vi "Read DSP Reset.vi"(2 "gen":refnum<class "niUSRP Tx DSP v2 FPGA.lvclass">) -> (4 "dsp reset":bool)   [LabVIEW 2025, in "niUSRP Tx DSP v2 FPGA.lvclass"]
doc: "this VI retrieves the dsp.reset signal as configured by the host. a maximum fanour constraint is placed on the signal so that our reset signal does not introduce high fanout nets that lead to Timing Errors (lower compile success rate). this VI should be used to read the reset signal so that all reset signals have the same pipelining applied to them. breaking the timing between resets across the fpga may create undesireable behavior."
uses:
  niUSRP Tx DSP v2 FPGA.lvclass
  niUSRP Tx DSP v2 FPGA.lvclass/niUSRP Tx DSP v2 FPGA.ctl
  <vilib>/rvi/DataTransferAndStorage/Container/Common/niFpgaContainerExecOnDevCompGetState.vi
  <vilib>/rvi/Emulation/niFpgaEmulationIsFPGAContextNoSignature.vi
  <vilib>/rvi/DataTransferAndStorage/Container/Common/niFpgaContainerGetUniqueNameForEmu.vi
  <vilib>/rvi/Memory/Memory_Emulation/niFpgaMemoryEmulationCacheClearOnFirstRun.vi
  <vilib>/rvi/Memory/Memory_Emulation/nirvimemoryEmulationManagerCache_MakeExclusive.vi
  <vilib>/rvi/Memory/Memory_Emulation/niFpgaMemoryEmulationValidateCache.vi
  <vilib>/rvi/Memory/Memory_Emulation/nirvimemoryEmulationManagerCache_InsertValue.vi
  <vilib>/Utility/error.llb/Clear Errors.vi
  <vilib>/rvi/Memory/Memory_Emulation/nirvimemoryEmulationManagerCache_ReleaseExclusive.vi
  <vilib>/rvi/Memory/Memory_Emulation/nirvimemoryEmulationManagerCache_GetValue.vi
  <vilib>/rvi/Memory/Memory_Emulation/nirvimemoryEmulationManagerCache_SetValue.vi
  <vilib>/rvi/Emulation/niFpgaProcessEmulError.vi
  <vilib>/rvi/Emulation/niFpgaSctlEmulationGetInTimedLoop.vi
  <vilib>/rvi/DataTransferAndStorage/Container/XNode/niFpgaContainer.xnode
  <vilib>/rvi/DataTransferAndStorage/Register/Emulation/niFpgaRegisterEmulationRefIn.vi
  <instrlib>/_niInstr/Basic Elements/v1/FPGA/niInstr Basic Elements v1 FPGA.lvlib
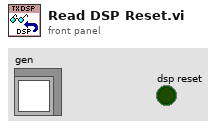
[diagram p1: front panel]
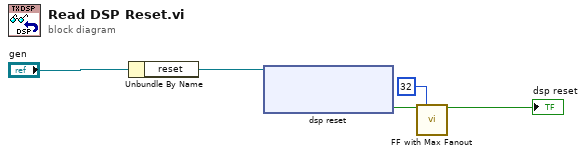
[diagram p0: block diagram]
diagram:
  n1 = Unbundle By Name("gen") -> ("reset"=w4:refnum<k21>)
  n2 = xnode "dsp reset"("Register In"=w4) -> ("Data"=w3:bool)  [unwired: 1 out]
  n3 = call <instrlib>:"FF with Max Fanout.vi"("cDataIn"=w3, "kMaxFanout"=u32 32) -> ("cDataOut"=→"dsp reset":bool)  [unwired: 13 in]
